vi "niRFSG Initiate.vi"(0 "instrument handle":refnum<k15>, 11 "error in":errorcluster {"code" format="%.0x"}) -> (4 "instrument handle out":refnum<k15>, 15 "error out":errorcluster {"code" format="%.0x"})   [LabVIEW 2014]
doc: "Initiates signal generation, causing the NI-RFSG device to leave the Configuration state or Committed state and enter the Generation state. If settings have not been committed to the device before you use this VI, they are committed by this VI. The operation returns when the RF output signal settles. To return to the Configuration state, use the niRFSG Abort VI.\n\n<B>Supported Devices</B>: NI 5611, NI 5644R/5645R/5646R, NI 5650/5651/5652/5654/5654 with NI 5696, NI 5670/5671/5672/5673/5673E, NI 5840"
uses:
  niRFSG.dll
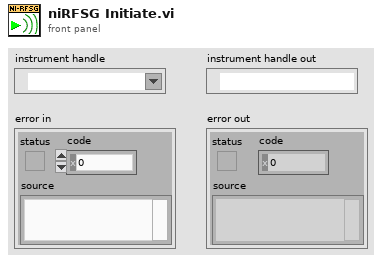
[diagram p1: front panel]
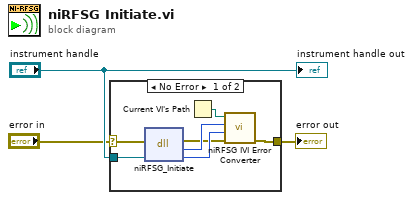
[diagram p0: block diagram]
diagram:
  n1 = case shown="No Error" "error in" {
    selector: "error in" -> [w5 w11]
    tunnel: "instrument handle" -> [w10 _]
    tunnel: [w9 w11] -> w1
    frame No Error {
      n2 = dll-call lib="niRFSG**.*" fn="niRFSG_Initiate"(error in=w5, "instrument handle"=w10) -> (error out=w4:errorcluster, "status"=w7:i32, "instrument handle"=w6:u32)  [unwired: 2 in, 1 out]
      n3 = Current VI's Path() -> (path=w8:path)
      n4 = call "niRFSG IVI Error Converter.vi"("error in"=w4, "instrument handle"=w6, "IVI error code"=w7, "path to VI"=w8) -> ("error out"=w9:errorcluster)  [unwired: 7 in]
    }
    frame Error {
    }
  }
  "error out" <- w1
  "instrument handle out" <- "instrument handle"
